vi "Harness - Action.vi"(8 "error in (no error)":errorcluster, 9 "BW icon in":T1, 10 "Color icon in":T1, 11 "Class":path=path "C:/git/labview-icon-editor/Sandbox/Class 2/_Class.lvclass") -> (0 "error out":errorcluster, 1 "BW icon out":T1, 2 "Color icon out":T1, 3 "Error code out":i32)   [LabVIEW 2021, in "IconEditorInterface.lvlib" / "IconEditorInterface.lvclass"]
uses:
  IconEditorInterface.lvclass
  <vilib>/picture/picture.llb/imagedata.ctl
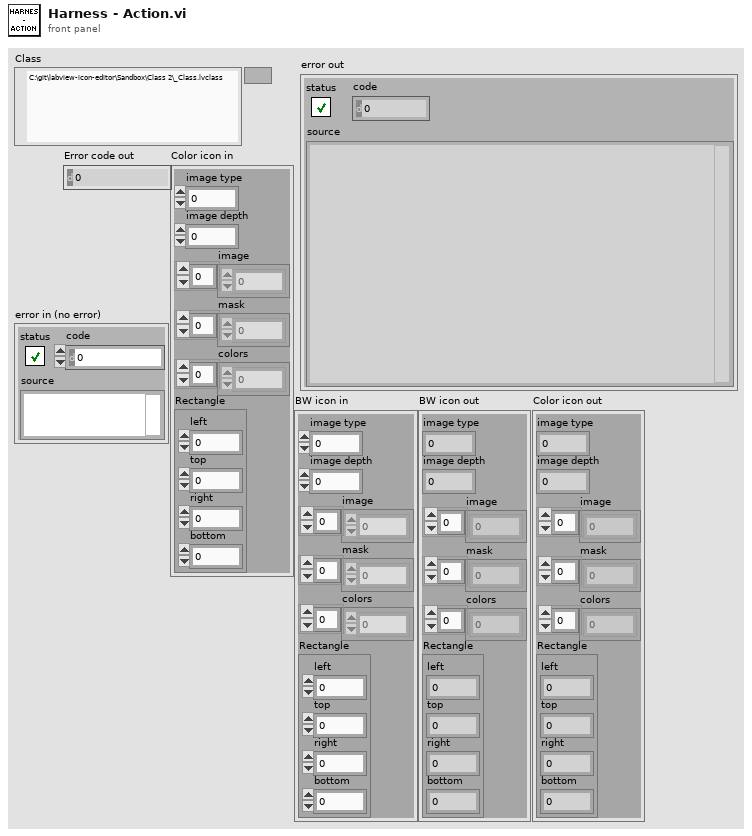
[diagram p1: front panel]
types:
  T1 = typedef "imagedata.ctl" = cluster{"image type":i32, "image depth":i32, "image":u8[], "mask":u8[], "colors":u32[], "Rectangle":cluster{"left":i16, "top":i16, "right":i16, "bottom":i16}}
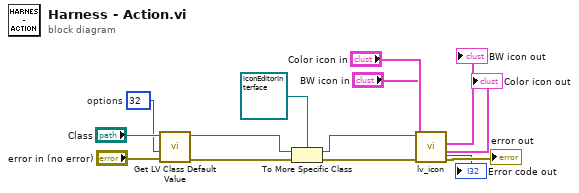
[diagram p0: block diagram]
diagram:
  w11 = u32 32  # options
  n1 = call <vilib>:"Get LV Class Default Value.vi"("error in (no error)"="error in (no error)", "options"=w11, "class path"="Class") -> ("error out"=w9:errorcluster, "object"=w14:refnum<class>)  [unwired: 7 in]
  n2 = To More Specific Class(target class=refnum<class "IconEditorInterface.lvclass"> refnum ("_IconEditorInterface.lvlib:_IconEditorInterface.lvclass"), reference=w14, error in=w9) -> (specific class reference=w6:refnum<class "IconEditorInterface.lvclass">, error out=w7:errorcluster)
  n3 = call-dynamic "lv_icon.vi"("error in (no error)"=w7, "BW icon in"="BW icon in", "Color icon in"="Color icon in", "_IconEditorInterface in"=w6) -> ("error out"=→"error out":errorcluster, "Color icon out"=→"Color icon out":T1, "BW icon out"=→"BW icon out":T1, "Error code out"=→"Error code out":i32)  [unwired: 3 in, 1 out]
